vi "jsonify with size.vi"   [LabVIEW 2015]
panel:
  # "Jsonify the input, prepending with 10 byte size string"
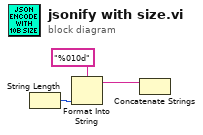
[diagram p0: block diagram]
diagram:
  n1 = String Length() -> (length=w3:i32)  [unwired: 1 in]
  n2 = Format Into String(format string="%010d", w3) -> (resulting string=w1:string)  [unwired: 2 in, 1 out]
  n3 = Concatenate Strings(w1) -> ()  [unwired: 1 in, 1 out]
